vi "LVFunction_Imop_Compute_ModalZonalWavefront.vi"(0 "HasoData":refnum<class "HasoData.lvclass">, 1 "HasoSlopes":refnum<class "HasoSlopes.lvclass">, 5 "ComputePhaseSet":refnum<class "ComputePhaseSet.lvclass">, 7 "Phase":refnum<class "Phase.lvclass">, 9 "ModalCoef.lvclass":refnum<class "ModalCoef.lvclass">, 11 "error constant":errorcluster) -> (3 "HasoSlopes (dup)":refnum<class "HasoSlopes.lvclass">, 4 "HasoData (dup)":refnum<class "HasoData.lvclass">, 6 "ComputePhaseSet (dup)":refnum<class "ComputePhaseSet.lvclass">, 8 "Phase":refnum<class "Phase.lvclass">, 10 "ModalCoef.lvclass (dup)":refnum<class "ModalCoef.lvclass">, 15 "error out":errorcluster)   [LabVIEW 2018]
doc: "Compute phase from slopes using both zonal and modal reconstruction.\n\n<B>ComputePhaseSetIn</B> : ComputePhaseSet object.\n<B>ComputePhaseSetOut</B> : ComputePhaseSet object.\n<B>HasoData</B> : HasoData object containing the input slopes.\n<B>ModalCoeffs</B> : ModalCoef object. Preferences are used as input, coefficients values are updated by the processing.\n<B>HasoSlopes</B> : HasoSlopes object containing the residual slopes.\n<B>Phase</B> : phase object. Phase values and steps are expressed in um."
uses:
  Classes/HasoData/HasoData.lvclass
  Classes/ComputePhaseSet/ComputePhaseSet.lvclass
  Classes/HasoSlopes/HasoSlopes.lvclass
  Classes/Phase/Phase.lvclass
  Classes/ModalCoef/ModalCoef.lvclass
  Classes/ModalCoef/LVClass_ModalCoef Read ModalCoef.vi
  Classes/HasoSlopes/LVClass_HasoSlopes Read HasoSlopes _ property.vi
  Classes/Phase/LVClasse_Phase Read SurfaceFloatWithPupil.vi
  Classes/ComputePhaseSet/LVClass_ComputePhaseSet Read ComputePhaseSet.vi
  Classes/HasoData/LVClass_HasoData Read HasoData - property.vi
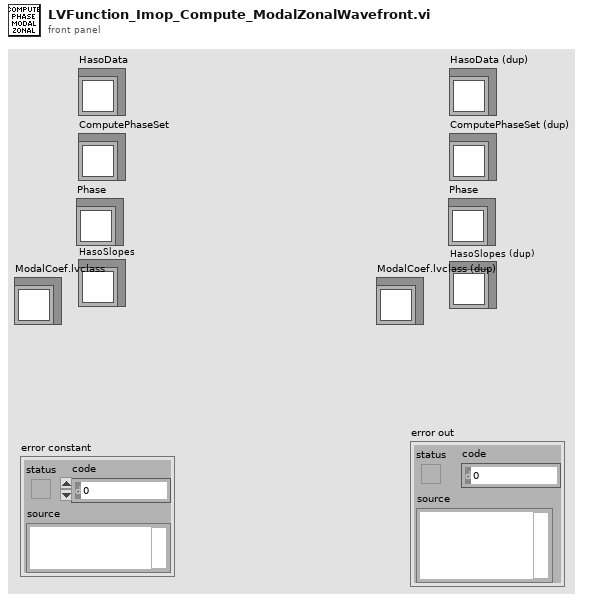
[diagram p1: front panel]
types:
  T1 = typedef "ClassID.ctl" = i64
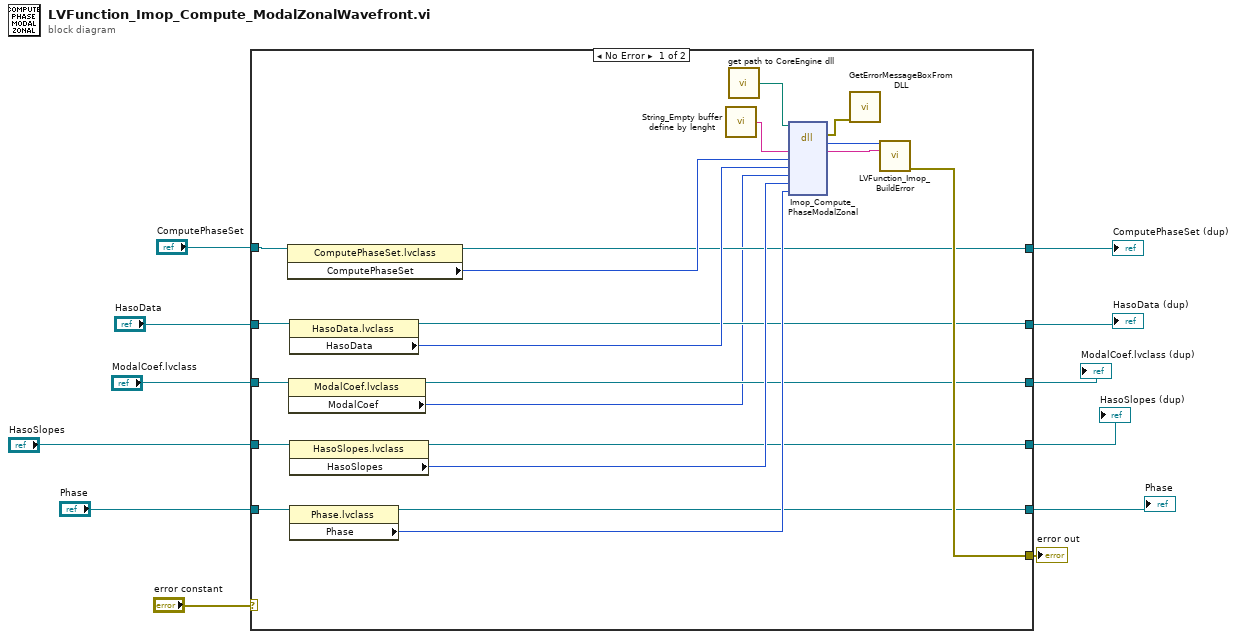
[diagram p0: block diagram]
diagram:
  n1 = case shown="No Error" "error constant" {
    selector: "error constant" -> [_ w39]
    tunnel: "HasoData" -> [w27 w37]
    tunnel: "ComputePhaseSet" -> [w26 w38]
    tunnel: [w28 w39] -> w11
    tunnel: "Phase" -> [w25 w36]
    tunnel: "HasoSlopes" -> [w21 w35]
    tunnel: [w19 w38] -> w7
    tunnel: [w18 w37] -> w6
    tunnel: [w17 w36] -> w5
    tunnel: [w16 w35] -> w3
    tunnel: "ModalCoef.lvclass" -> [w15 w34]
    tunnel: [w14 w34] -> w1
    frame No Error {
      n2 = property class="ComputePhaseSet.lvclass"(reference=w26) -> (reference out=w19:refnum<class "ComputePhaseSet.lvclass">, "ComputePhaseSet"=w23:T1)  [unwired: 1 in, 1 out]
      n3 = property class="ModalCoef.lvclass"(reference=w15) -> (reference out=w14:refnum<class "ModalCoef.lvclass">, "ModalCoef"=w13:T1)  [unwired: 1 in, 1 out]
      n4 = property class="HasoData.lvclass"(reference=w27) -> (reference out=w18:refnum<class "HasoData.lvclass">, "HasoData"=w24:T1)  [unwired: 1 in, 1 out]
      n5 = property class="HasoSlopes.lvclass"(reference=w21) -> (reference out=w16:refnum<class "HasoSlopes.lvclass">, "HasoSlopes"=w20:T1)  [unwired: 1 in, 1 out]
      n6 = property class="Phase.lvclass"(reference=w25) -> (reference out=w17:refnum<class "Phase.lvclass">, "Phase"=w22:T1)  [unwired: 1 in, 1 out]
      n7 = call "String_Empty buffer define by lenght.vi"() -> ("Empty buffer"=w31:string)  [unwired: 1 in]
      n8 = call "get path to CoreEngine dll.vi"() -> ("path to wavekit library"=w30:path)  [unwired: 14 in, 1 out]
      n9 = dll-call lib="D:/FLE/0.Code/CoreEngine4_Suite/LV2011_interface/DLLs/c_interface_vc100.dll" fn="Imop_Compute_PhaseModalZonal"(path in=w30, "message"=w31, "ComputePhaseSet"=w23, "HasoData"=w24, "ModalCoeffs"=w13, "ResidualHasoSlopes"=w20, "phase"=w22) -> (error out=w29:errorcluster, "return type"=w33:i32, "message"=w32:string)  [unwired: 7 in, 1 out]
      n10 = call "GetErrorMessageBoxFromDLL.vi"("error IN"=w29) -> ()  [unwired: 10 in, 1 out]
      n11 = call "LVFunction_Imop_BuildError.vi"("code"=w33, "String to Prepend to source (\"\")"=w32) -> ("error out"=w28:errorcluster)  [unwired: 13 in]
    }
    frame Error {
    }
  }
  "error out" <- w11
  "ComputePhaseSet (dup)" <- w7
  "HasoData (dup)" <- w6
  "Phase" <- w5
  "HasoSlopes (dup)" <- w3
  "ModalCoef.lvclass (dup)" <- w1
